vi "MidbrainBehaviorEngine.vi"(11 "Forebrain Cmd":T2) -> (0 "Cluster":T1={"P-WallFollow"=TRUE, "AvoidWall"=TRUE, "Seek IR"=TRUE, " Push Home"=TRUE, "Go Home"=TRUE}, 3 "VelCom":dbl)   [LabVIEW 2011]
doc: "This sub VI takes the commanded mission velocity and robot behavior from the Forebrain and activates the appropriate Midbrain subbehaviors to cary it out."
uses:
  ForebrainCmd.ctl
  Behaviour.ctl
  MidbrainBehaviour.ctl
panel:
  # "This subVI takes the current desired robot\nvelocity andoverall  behavior from the Forebrain\nand activates the appropriate Midbrain sub-behaviors\nto carry it out"
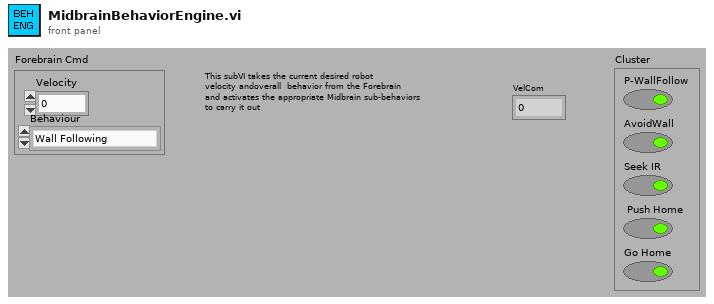
[diagram p1: front panel]
types:
  T1 = typedef "MidbrainBehaviour.ctl" = cluster{"P-WallFollow":bool, "AvoidWall":bool, "Seek IR":bool, " Push Home":bool, "Go Home":bool}
  T2 = typedef "ForebrainCmd.ctl" = cluster{"Velocity":dbl, "Behaviour":T3}
  T3 = typedef "Behaviour.ctl" = enum16{"Wall Following", "Open Transit", "Find Barge", "Push Barge", "Go Home"}
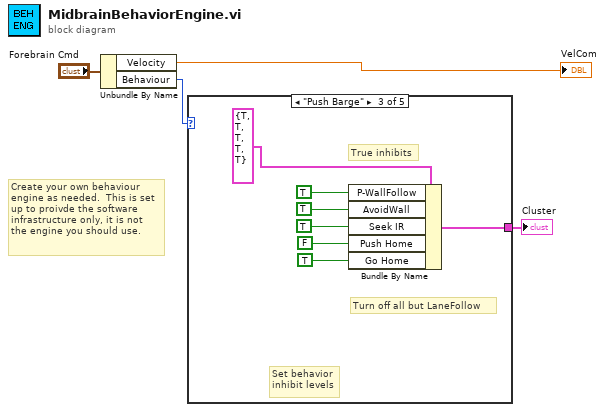
[diagram p0: block diagram]
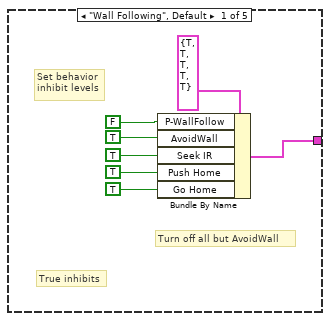
[diagram p2: hidden frame]
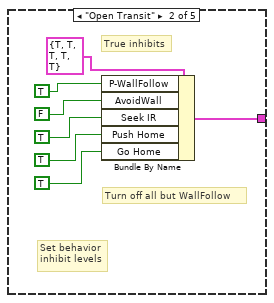
[diagram p3: hidden frame]
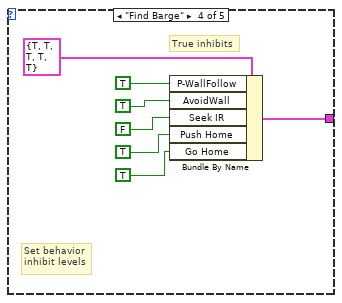
[diagram p4: hidden frame]
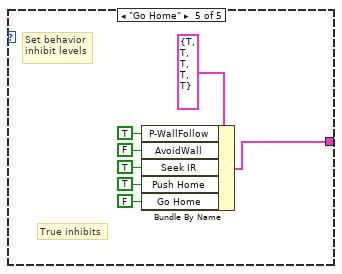
[diagram p5: hidden frame]
diagram:
  # "Create your own behaviour\nengine as needed.  This is set\nup to proivde the software \ninfrastructure only, it is not\nthe engine you should use."
  n1 = Unbundle By Name("Forebrain Cmd") -> ("Velocity"=→"VelCom":dbl, "Behaviour"=w2:T3)
  n2 = case shown="\"Push Barge\"" w2 {
    tunnel: [w7 w13 w20 w27 w38] -> w1
    frame "Wall Following", Default {
      # "True inhibits"
      # "Set behavior\ninhibit levels"
      # "Turn off all but AvoidWall"
      n3 = Bundle By Name(cluster=T1 {"P-WallFollow"=TRUE, "AvoidWall"=TRUE, "Seek IR"=TRUE, " Push Home"=TRUE, "Go Home"=TRUE}, "P-WallFollow"=FALSE ("LaneFollow"), "AvoidWall"=TRUE ("WallFollow"), "Seek IR"=TRUE ("Wander"), "Push Home"=TRUE ("AvoidWall"), "Go Home"=TRUE ("AvoidWall")) -> (w7:T1)
    }
    frame "Open Transit" {
      # "True inhibits"
      # "Set behavior\ninhibit levels"
      # "Turn off all but WallFollow"
      n4 = Bundle By Name(cluster=T1 {"P-WallFollow"=TRUE, "AvoidWall"=TRUE, "Seek IR"=TRUE, " Push Home"=TRUE, "Go Home"=TRUE}, "P-WallFollow"=TRUE ("LaneFollow"), "AvoidWall"=FALSE ("WallFollow"), "Seek IR"=TRUE ("Wander"), "Push Home"=TRUE ("AvoidWall"), "Go Home"=TRUE ("AvoidWall")) -> (w13:T1)
    }
    frame "Push Barge" {
      # "True inhibits"
      # "Set behavior\ninhibit levels"
      # "Turn off all but LaneFollow"
      n5 = Bundle By Name(cluster=T1 {"P-WallFollow"=TRUE, "AvoidWall"=TRUE, "Seek IR"=TRUE, " Push Home"=TRUE, "Go Home"=TRUE}, "P-WallFollow"=TRUE ("LaneFollow"), "AvoidWall"=TRUE ("WallFollow"), "Seek IR"=TRUE ("Wander"), "Push Home"=FALSE ("AvoidWall"), "Go Home"=TRUE ("AvoidWall")) -> (w20:T1)
    }
    frame "Find Barge" {
      # "True inhibits"
      # "Set behavior\ninhibit levels"
      n6 = Bundle By Name(cluster=T1 {"P-WallFollow"=TRUE, "AvoidWall"=TRUE, "Seek IR"=TRUE, " Push Home"=TRUE, "Go Home"=TRUE}, "P-WallFollow"=TRUE ("LaneFollow"), "AvoidWall"=TRUE ("WallFollow"), "Seek IR"=FALSE ("Wander"), "Push Home"=TRUE ("AvoidWall"), "Go Home"=TRUE ("AvoidWall")) -> (w27:T1)
    }
    frame "Go Home" {
      # "True inhibits"
      # "Set behavior\ninhibit levels"
      n7 = Bundle By Name(cluster=T1 {"P-WallFollow"=TRUE, "AvoidWall"=TRUE, "Seek IR"=TRUE, " Push Home"=TRUE, "Go Home"=TRUE}, "P-WallFollow"=TRUE, "AvoidWall"=FALSE, "Seek IR"=TRUE, "Push Home"=TRUE ("Find Gap"), "Go Home"=FALSE ("Wander")) -> (w38:T1)
    }
  }
  "Cluster" <- w1
